vi "Validate Project API.vi"   [LabVIEW 2011]
uses:
  VI Tester Project API.lvlib
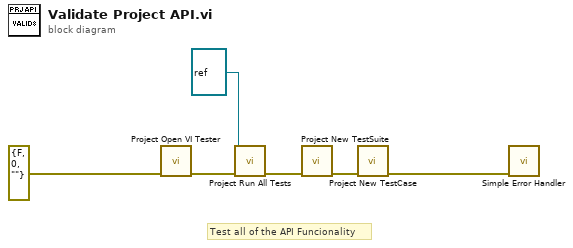
[diagram p0: block diagram]
diagram:
  # "Test all of the API Funcionality"
  n1 = call "Project Open VI Tester.vi"("error in (no error)"=errorcluster {"status"=FALSE, "code"=0, "source"=""}) -> ("error out"=w2:errorcluster)  [unwired: 10 in]
  n2 = call "Project Run All Tests.vi"("error in (no error)"=w2, "VI Tester reference"=refnum<vi> refnum) -> ("error out"=w5:errorcluster)  [unwired: 9 in]
  n3 = call "Project New TestSuite.vi"("error in (no error)"=w5) -> ("error out"=w4:errorcluster)  [unwired: 10 in]
  n4 = call "Project New TestCase.vi"("error in (no error)"=w4) -> ("error out"=w3:errorcluster)  [unwired: 10 in]
  n5 = call <vilib>:"Simple Error Handler.vi"("error in (no error)"=w3) -> ()  [unwired: 4 in, 5 out]
